vi "Read Pressure Range.vi"(7 "Channel (0: Channel A)":u16(ring) items=["Channel A", "Channel B"], 8 "error in (no error)":errorcluster, 11 "BH Druck PACE Series in":refnum<class "BH Druck PACE Series.lvclass">) -> (0 "error out":errorcluster, 1 "-FS Range/mbar":dbl, 2 "+FS Range/mbar":dbl, 3 "BH Druck PACE Series out":refnum<class "BH Druck PACE Series.lvclass">, 4 "Range":string)   [LabVIEW 2022 SP3, in "BH Druck PACE Series.lvclass"]
uses:
  BH Druck PACE Series.lvclass
  BH Druck PACE Series.lvclass/BH Druck PACE Series.ctl
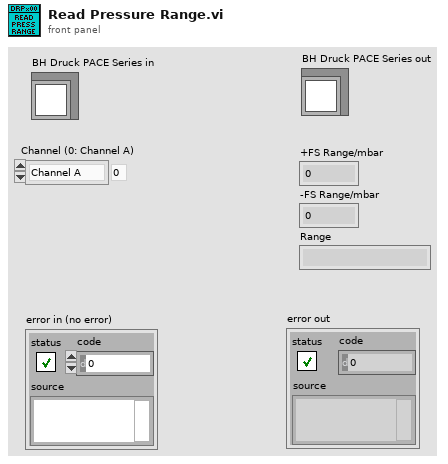
[diagram p1: front panel]
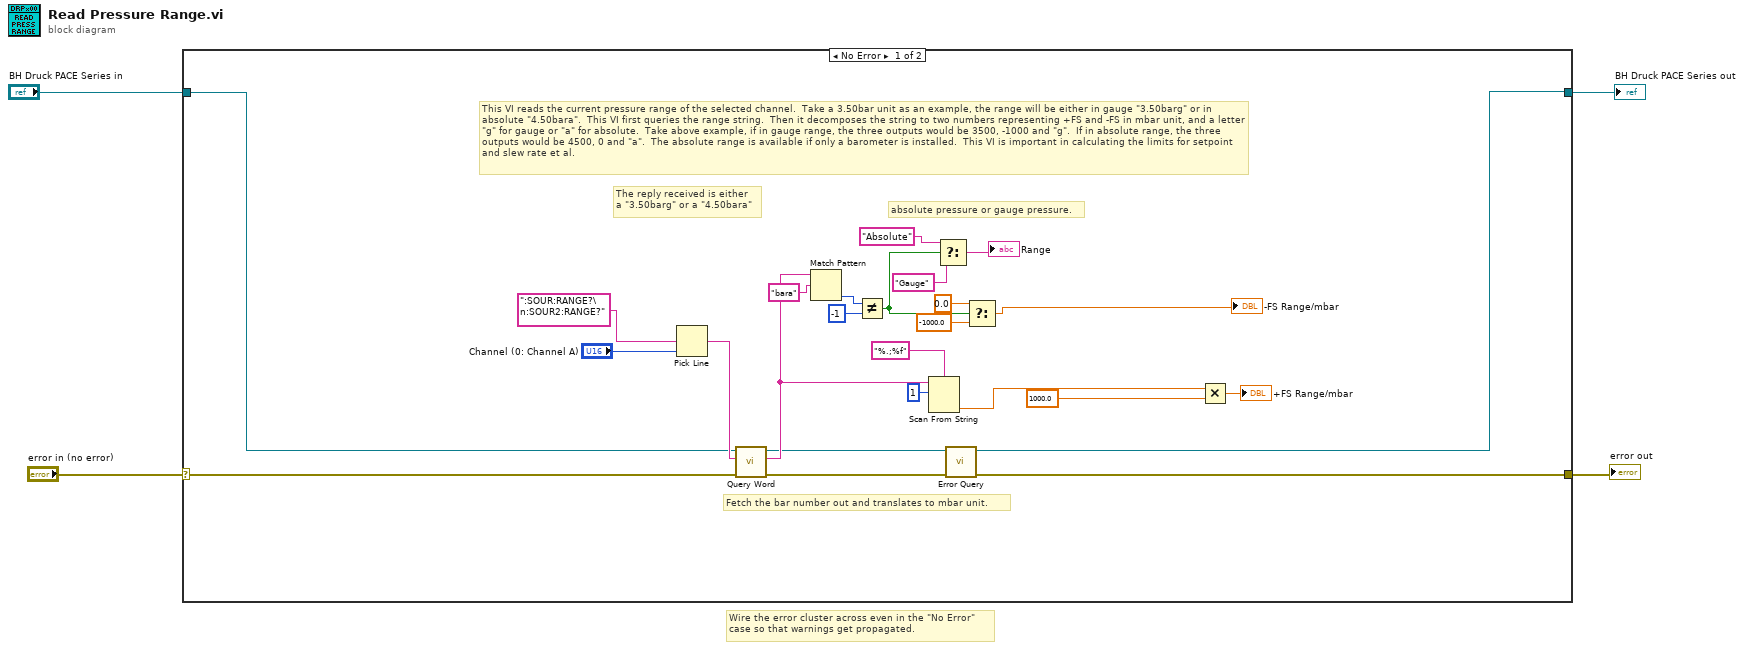
[diagram p0: block diagram]
diagram:
  # "Wire the error cluster across even in the \"No Error\"\ncase so that warnings get propagated."
  n1 = case shown="No Error" "error in (no error)" {
    selector: "error in (no error)" -> [w9 w31]
    tunnel: [w6 w31] -> w3
    tunnel: [w5 w30] -> w1
    tunnel: "BH Druck PACE Series in" -> [w8 w30]
    frame No Error {
      # "This VI reads the current pressure range of the selected channel.  Take a 3.50bar unit as an example, the range will be either in gauge \"3.50barg\" or in absolute \"4.50bara\".  This VI first queries the range string.  Then it decomposes the string to two numbers representing +FS and -FS in mbar unit, and a letter \"g\" for gauge or \"a\" for absolute.  Take above example, if in gauge range, the three outputs would be 3500, -1000 and \"g\".  If in absolute range, the three outputs would be 4500, 0 and \"a\".  The absolute range is available if only a barometer is installed.  This VI is important in calculating the limits for setpoint and slew rate et al."
      # "absolute pressure or gauge pressure."
      # "Fetch the bar number out and translates to mbar unit."
      # "The reply received is either \na \"3.50barg\" or a \"4.50bara\""
      n2 = Pick Line(multi-line string=":SOUR:RANGE?\n:SOUR2:RANGE?", line index="Channel (0: Channel A)") -> (output string=w20:string)  [unwired: 1 in]
      n3 = call-dynamic "Query Word.vi"("error in (no error)"=w9, "Query String"=w20, "BH Druck PACE Series in"=w8) -> ("error out"=w24:errorcluster, "String Result"=w25:string, "BH Druck PACE Series out"=w7:refnum<class "BH Druck PACE Series.lvclass">)  [unwired: 6 in]
      n4 = Match Pattern(string=w25, regular expression="bara") -> (offset past match=w26:i32)  [unwired: 1 in, 3 out]
      n5 = Not Equal?(x=w26, y=-1) -> (x != y?=w28:bool)
      n6 = Scan From String(format string="%.;%f", input string=w25, initial scan location=u32 1) -> (output 1=w22:dbl)  [unwired: 2 in, 3 out]
      n7 = Select(t="Absolute", s=w28, f="Gauge") -> (s? t:f=→"Range":string)
      n8 = call-dynamic "Error Query.vi"("error in (no error)"=w24, "BH Druck PACE Series in"=w7) -> ("error out"=w6:errorcluster, "BH Druck PACE Series out"=w5:refnum<class "BH Druck PACE Series.lvclass">)  [unwired: 8 in]
      n9 = Select(t=0.0, s=w28, f=-1000.0) -> (s? t:f=→"-FS Range/mbar":dbl)
      n10 = Multiply(x=w22, y=1000.0) -> (x*y=→"+FS Range/mbar":dbl)
    }
    frame Error {
    }
  }
  "error out" <- w3
  "BH Druck PACE Series out" <- w1
